vi "Read Subscriber List.vi"(8 "error in":errorcluster, 10 "Topic Name":string, 11 "Broker in":refnum<class "Broker.lvclass">) -> (0 "error out":errorcluster, 1 "Subscriber List":string[](array[string]), 2 "Topic Name Out":string, 3 "Broker out":refnum<class "Broker.lvclass">)   [LabVIEW 2014, in "Broker.lvclass"]
uses:
  Broker.lvclass
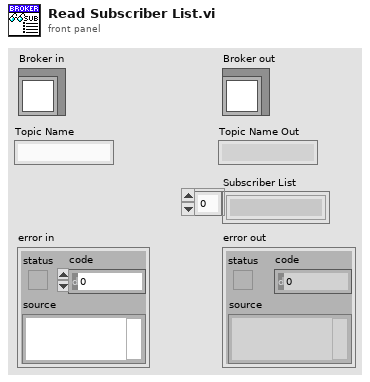
[diagram p1: front panel]
types:
  T1 = typedef "Topic Ref.ctl" = cluster{"Name":string, "Path":path, "Subscribers":string[]}
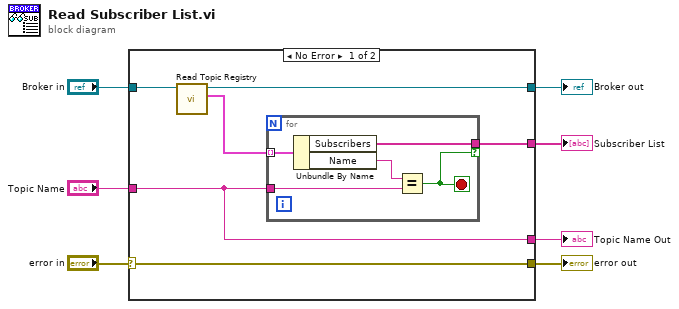
[diagram p0: block diagram]
diagram:
  n1 = case shown="No Error" "error in" {
    selector: "error in" -> [w13 w21]
    tunnel: [w13 w21] -> w6
    tunnel: [w9 w20] -> w4
    tunnel: "Broker in" -> [w12 w20]
    tunnel: "Topic Name" -> [w10 w19]
    tunnel: [w11 _] -> w2
    tunnel: [w10 w19] -> w1
    frame No Error {
      n2 = call-dynamic "Read Topic Registry.vi"("Broker in"=w12) -> ("Topic Registry"=w8:T1[], "Broker out"=w9:refnum<class "Broker.lvclass">)  [unwired: 8 in, 1 out]
      n3 = for {
        tunnel: w8 -> [w16] mode=indexing
        tunnel: w10 -> [w18]
        tunnel: [w15] -> w11 if=w14
        stop <- w14 stop-if-true
        n4 = Unbundle By Name(w16) -> ("Subscribers"=w15:string[], "Name"=w17:string)
        n5 = Equal?(x=w17, y=w18) -> (x = y?=w14:bool)
      }
    }
    frame Error {
    }
  }
  "error out" <- w6
  "Broker out" <- w4
  "Subscriber List" <- w2
  "Topic Name Out" <- w1
